vi "Measuring Complete - AndreTec-2.vi"() -> ()   [LabVIEW 2014]
doc: "André Romero - 2016\nandretec@ifsc.usp.br\nIFSC - USP"
uses:
  Program Files/National Instruments/LabVIEW 2014/examples/Instrument IO/Serial/support/Serial - Settings.ctl
  <vilib>/Analysis/Matrix/Datatypes/RealMatrix.ctl
  C:/Users/user/Documents/Andre/AutoLAB/Autolab SDK 1.11/EcoChemie.Autolab.Sdk.dll
  EcoChemie.Autolab.Sdk.dll
  <vilib>/Instr/_visa.llb/VISA Configure Serial Port (Instr).vi
  <vilib>/Utility/file.llb/Write To Spreadsheet File (DBL).vi
  <vilib>/Analysis/Matrix/NI_Matrix.lvlib
panel:
  out "Numeric":i32=27341680
  in  "Start Measurement":bool
  out "Sensor":i32=1
  out "error out":errorcluster={"status"=TRUE, "code"=-1073807343, "source"="Property Node (arg 1) in VISA Configure Serial Port (Instr).vi->Measuring Complete - AndreTec-2.vi"}
  out "VISA resource name out":refnum<visa-resource-name>="COM3"
  in  "N. Sensors":i32=3 min=1 max=8
  in  "VISA resource name":refnum<visa-resource-name>="COM5"
  out "Measured data 2":cluster{dbl[], dbl[]}(graph)
  out "Points":i32=478
  in  "Abort":bool
  in  "Y axis Signal":string(combo)="WE(1).Current"
  in  "X axis Signal":string(combo)="WE(1).Potential"
  out "Measured data":cluster{"Y":dbl[], "Y":dbl[]}[](graph)
  out "X axis value":dbl=-1.1810302734375e-08
  out "Y axis value":dbl=3.0517578124972244e-06
  out "Measurement active":bool
  out "Blacklisted Commands detected":bool
  in  "Load Procedure":path=path "C:/Users/user/Documents/My Procedures 1.11/Procedures/bla.nox"
  out "Autolab Connected":bool
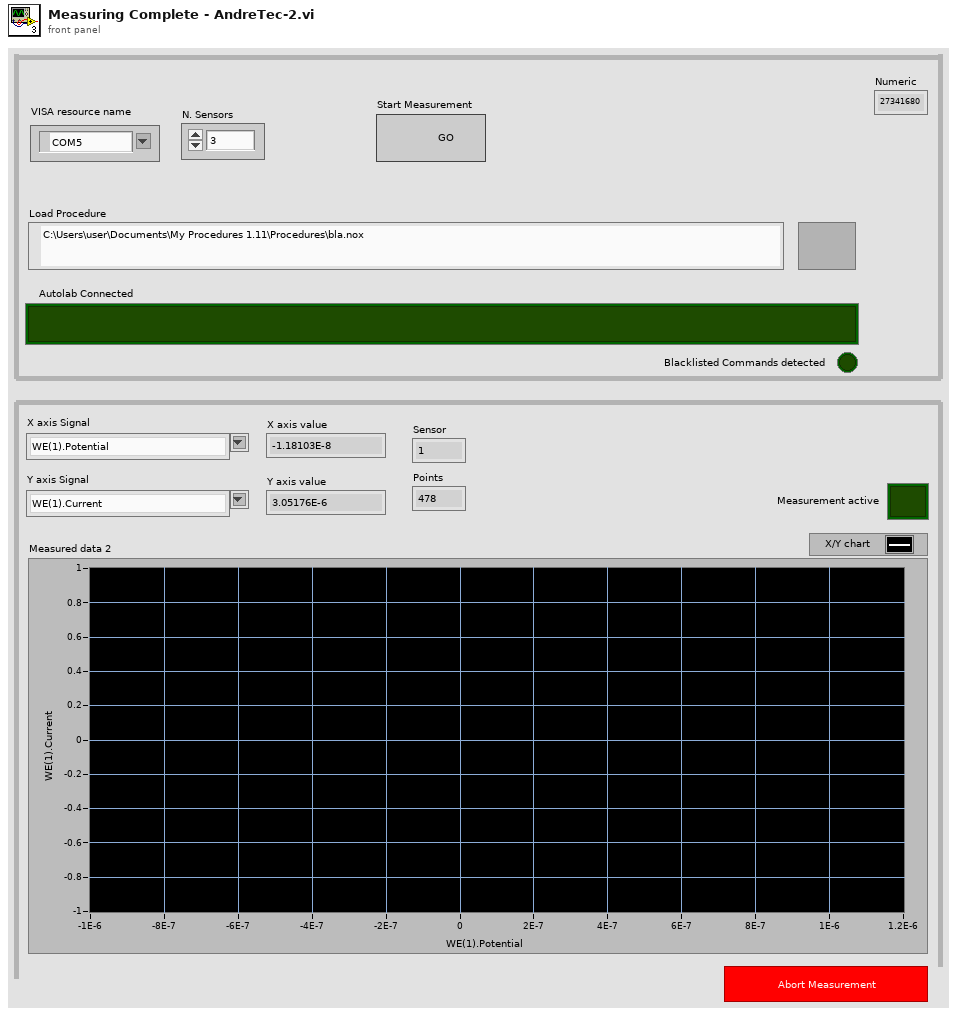
[diagram p1: front panel]
types:
  T1 = typedef "NI_Matrix.lvlib/RealMatrix.ctl" = dbl[][]
  T2 = typedef "Serial - Settings.ctl" = cluster{"baud rate":u32, "data bits":u16, "parity":enum16{"None", "Odd", "Even", "Mark", "Space"}, "stop bits":u16, "flow control":u16}
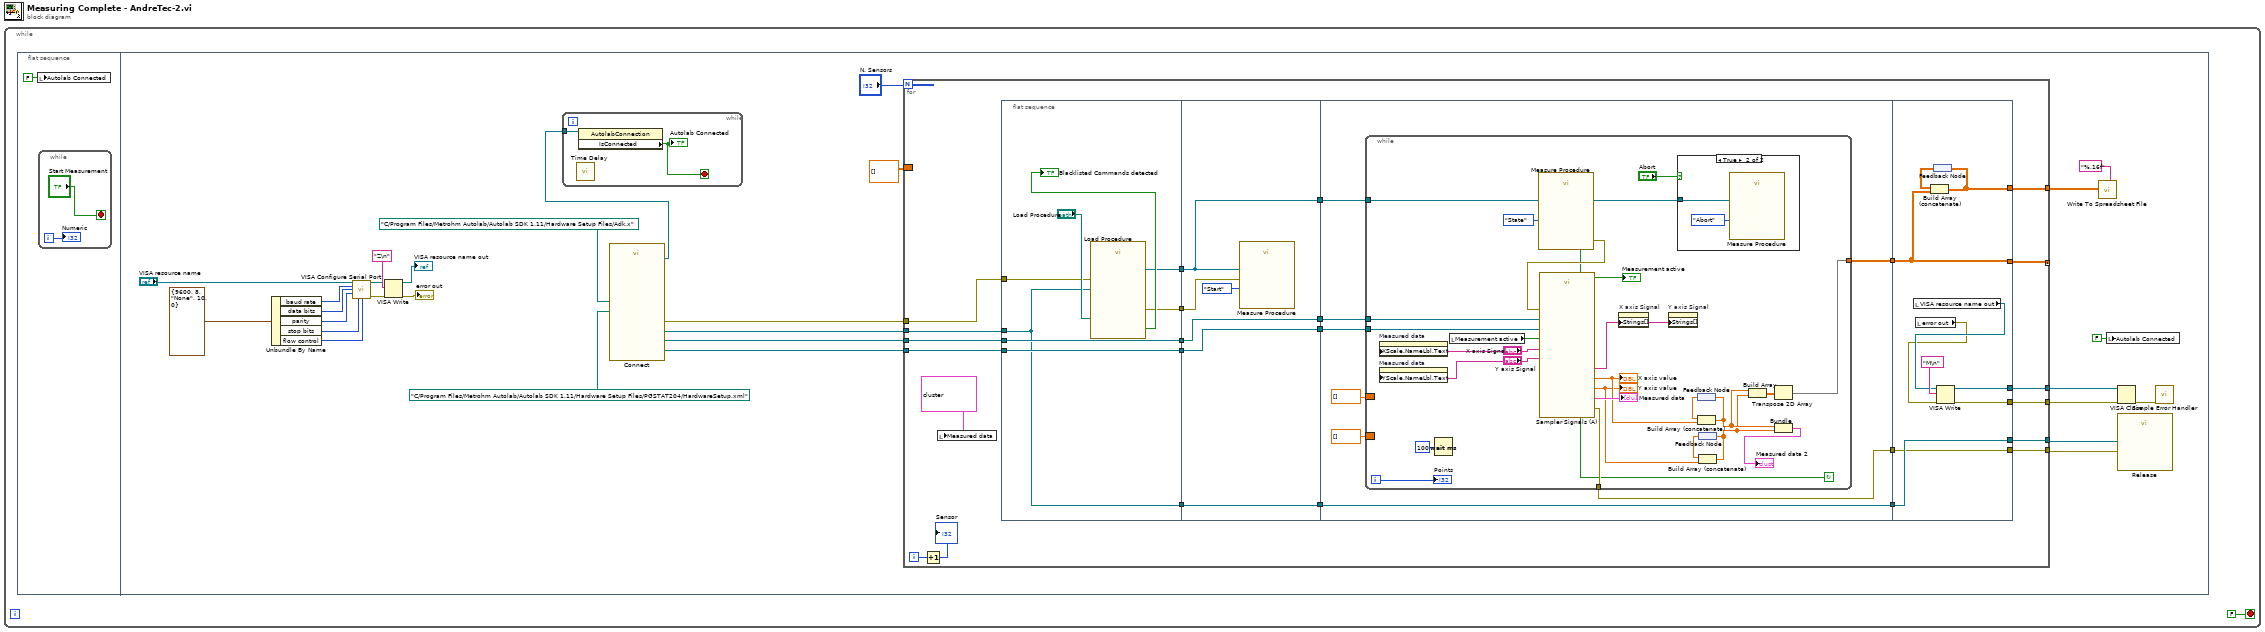
[diagram p0: block diagram]
diagram:
  n1 = while {
    stop <- FALSE stop-if-true
    n2 = flat-sequence {
      frame #0 {
        n3 = local write "Autolab Connected"(FALSE ("Autolab Connected")) -> ()
        n4 = while {
          i -> [w3]
          stop <- "Start Measurement" stop-if-true
          "Numeric" <- w3
        }
      }
      frame #1 {
        n5 = Unbundle By Name(T2 {"baud rate"=9600, "data bits"=8, "parity"=enum."None", "stop bits"=10, "flow control"=0} ("Serial Settings")) -> ("baud rate"=w29:u32, "data bits"=w30:u16, "parity"=w31:enum16{"None", "Odd", "Even", "Mark", "Space"}, "stop bits"=w32:u16, "flow control"=w33:u16)
        n6 = call-poly "VISA Configure Serial Port"("VISA resource name"="VISA resource name", "baud rate (9600)"=w29, "data bits (8)"=w30, "parity (0:none)"=w31, "stop bits (10: 1 bit)"=w32, "flow control (0:none)"=w33) -> ("VISA resource name out"=w12:refnum<visa-resource-name>, "error out"=w11:errorcluster)  [unwired: 3 in, 5 out]
        n7 = VISA Write(VISA resource name=w12, write buffer="Z\n" ("Command"), error in (no error)=w11) -> (VISA resource name out=→"VISA resource name out":refnum<visa-resource-name>, error out=→"error out":errorcluster)  [unwired: 1 out]
        n8 = call "Connect.vi"("Embedded Exe File"=path "C:/Program Files/Metrohm Autolab/Autolab SDK 1.11/Hardware Setup Files/Adk.x", "Hardware Setup File"=path "C:/Program Files/Metrohm Autolab/Autolab SDK 1.11/Hardware Setup Files/PGSTAT204/HardwareSetup.xml") -> ("Sampler"=w15:refnum<k24>, "AutolabConnection"=w18:refnum<k24>, "instrument"=w16:refnum<k24>, "Ei"=w14:refnum<k24>, "error out"=w17:errorcluster)  [unwired: 1 in, 8 out]
        n9 = while {
          tunnel: w18 -> [w34]
          stop <- w35 stop-if-true
          n10 = call "Time Delay"() -> ()  [unwired: 2 in, 10 out]
          n11 = property class="AutolabConnection"(reference=w34) -> ("IsConnected"=w35:bool)  [unwired: 1 in, 2 out]
          "Autolab Connected" <- w35
        }
        n12 = for {
          N: "N. Sensors" -> [_]
          tunnel: [w49] -> w26
          tunnel: [w48] -> w25
          tunnel: [w47] -> w22
          tunnel: [w46] -> w21
          tunnel: w17 -> [w45]
          tunnel: w16 -> [w44]
          tunnel: w15 -> [w43]
          tunnel: w14 -> [w42]
          tunnel: [w40] -> _ mode=concatenating
          tunnel: [w38] -> w8
          border: T1 [] ("Real Matrix") -> [_]
          i -> [w37]
          n13 = Increment(x=w37) -> (x+1=→"Sensor":i32)
          n14 = local write "Measured data"(cluster{"Y":dbl[], "Y":dbl[]}[] [{"Y"=array[2393 elements], "Y"=array[2393 elements]}] ("Measured data")) -> ()
          n15 = flat-sequence {
            tunnel: [w66] -> w60
            tunnel: [w65] -> w59
            tunnel: [w63] -> w58
            tunnel: [w62] -> w57
            tunnel: [w61] -> w56
            tunnel: w44 -> [w61]
            tunnel: w45 -> [w64]
            tunnel: w43 -> [w63]
            tunnel: w42 -> [w62]
            tunnel: w60 -> [w72]
            tunnel: w59 -> [w73]
            tunnel: [w72] -> w55
            tunnel: w58 -> [w71]
            tunnel: w57 -> [w70]
            tunnel: [w71] -> w54
            tunnel: [w70] -> w53
            tunnel: [w69] -> w52
            tunnel: w56 -> [w69]
            tunnel: w55 -> [w82]
            tunnel: w54 -> [w81]
            tunnel: w53 -> [w80]
            tunnel: w52 -> [w79]
            tunnel: [w79] -> w51
            tunnel: [w78] -> w50
            tunnel: [w77] -> w39
            tunnel: w51 -> [w118]
            tunnel: w50 -> [w117]
            tunnel: [w118] -> w49
            tunnel: [w117] -> w48
            tunnel: [w113] -> w47
            tunnel: [w112] -> w46
            tunnel: [w111] -> w40
            tunnel: w39 -> [w111]
            tunnel: [w109] -> w38
            frame #0 {
              n16 = call "Load Procedure.vi"("error in (no error)"=w64, "Procedure"="Load Procedure", "Instrument"=w61) -> ("error out"=w65:errorcluster, "Contains"=→"Blacklisted Commands detected":bool, "LoadProcedure"=w66:refnum<k24>)  [unwired: 6 out]
            }
            frame #1 {
              n17 = call "Measure Procedure.vi"("error in"=w73, "Request for procedure"=enum16{"State", "Save", "Abort", "Start"}."Start", "LoadProcedure"=w72) -> ()  [unwired: 1 in, 8 out]
            }
            frame #2 {
              n18 = while {
                tunnel: w82 -> [w97]
                tunnel: w81 -> [w99]
                tunnel: w80 -> [w98]
                tunnel: [w88] -> w78
                tunnel: [w83] -> w77
                border: dbl[] [] -> [_]
                border: dbl[] [] -> [_]
                i -> [w94]
                stop <- w87 continue-if-true
                n19 = property on="Measured data" class="XYGraph (strict)"("XScale.NameLbl.Text"="X axis Signal") -> ()  [unwired: 2 in, 2 out]
                n20 = property on="Measured data" class="XYGraph (strict)"("YScale.NameLbl.Text"="Y axis Signal") -> ()  [unwired: 2 in, 2 out]
                n21 = Wait (ms)(milliseconds to wait=u32 100) -> ()  [unwired: 1 out]
                n22 = local read "Measurement active"() -> (w101:bool)
                n23 = call "Measure Procedure.vi"("Request for procedure"=enum16{"State", "Save", "Abort", "Start"}."State", "LoadProcedure"=w97) -> ("error out"=w102:errorcluster, "IsMeasuring"=w87:bool)  [unwired: 2 in, 6 out]
                "Measurement active" <- w87
                n24 = call "Sampler Signals (A).vi"("IsMeasuring"=w101, "EI"=w98, "Sampler"=w99, "Signal X"="X axis Signal", "Signal Y"="Y axis Signal", "error in"=w102) -> ("X"=w92:dbl, "Y"=w90:dbl, "XY Graph"=→"Measured data":cluster{"Y":dbl[], "Y":dbl[]}[], "GetSignals"=w104:string[], "error out"=w88:errorcluster)  [unwired: 4 in, 1 out]
                "Y axis value" <- w90
                "X axis value" <- w92
                n25 = property on="X axis Signal" class="CmbBox"("Strings[]"=w104) -> ()  [unwired: 2 in, 2 out]
                n26 = property on="Y axis Signal" class="CmbBox"("Strings[]"=w104) -> ()  [unwired: 2 in, 2 out]
                n27 = case shown="True" "Abort" {
                  tunnel: w97 -> [_ w107]
                  frame False {
                  }
                  frame True {
                    n28 = call "Measure Procedure.vi"("Request for procedure"=enum16{"State", "Save", "Abort", "Start"}."Abort", "LoadProcedure"=w107) -> ()  [unwired: 2 in, 8 out]
                  }
                }
                n29 = feedback #1() -> (w93:dbl[])
                n30 = Build Array (concatenate)(w93, w92) -> (w85:dbl[])
                n31 = feedback-in #1(w85) -> ()
                n32 = feedback #2() -> (w91:dbl[])
                n33 = Build Array (concatenate)(w91, w90) -> (w84:dbl[])
                n34 = feedback-in #2(w84) -> ()
                n35 = Build Array(w85, w84) -> (w86:dbl[][])
                n36 = Transpose 2D Array(2D array=w86) -> (transposed array=w83:dbl[][])
                n37 = Bundle(w85, w84) -> (→"Measured data 2":cluster{dbl[], dbl[]})  [unwired: 1 in]
                "Points" <- w94
              }
            }
            frame #3 {
              n38 = local read "VISA resource name out"() -> (w115:refnum<visa-resource-name>)
              n39 = local read "error out"() -> (w114:errorcluster)
              n40 = feedback #3() -> (w110:T1)
              n41 = Build Array (concatenate)(w110, w111) -> (w109:T1)
              n42 = feedback-in #3(w109) -> ()
              n43 = VISA Write(VISA resource name=w115, write buffer="M\n" ("Command"), error in (no error)=w114) -> (VISA resource name out=w113:refnum<visa-resource-name>, error out=w112:errorcluster)  [unwired: 1 out]
            }
          }
        }
        n44 = call-poly <vilib>:"Write To Spreadsheet File.vi"("format (%.3f)"="%.16f", "2D data"=w8) -> ()  [unwired: 6 in, 1 out]
        n45 = local write "Autolab Connected"(FALSE ("Autolab Connected")) -> ()
        n46 = call "Release.vi"("error in (no error)"=w25, "Instrument"=w26) -> ()  [unwired: 1 in, 9 out]
        n47 = VISA Close(VISA resource name=w22, error in (no error)=w21) -> (error out=w23:errorcluster)
        n48 = call <vilib>:"Simple Error Handler.vi"("error in (no error)"=w23) -> ()  [unwired: 1 in, 8 out]
      }
    }
  }
